vi "Robot Global Data.vi"() -> ()   [LabVIEW 2011]
doc: "This global VI can contain as many global variables as you need. Place a control on the panel, give it a good name. To read or write to it from a VI, drag the icon to the diagram of that VI. You can also drag from the project. Click on the node to change which global you access. You shouldn't have multiple locations writing to a global or it will cause a race-condition."
uses:
  <vilib>/Rock Robotics/WPI/Camera/WPI_CameraImageSize.ctl
panel:
  out "AUTO ON":bool
  out "is in auto":bool
  out "Target Locked":bool
  in  "Xerror":dbl=0.1
  in  "AUTO ON int":u8
  in  "teleop on":u8
  in  "Selected Distance":dbl
  in  "Distance":dbl
  in  "Elevator Button Prev":u8
  in  "Elevator Toggle":u8
  in  "LED toggle rate (ms)":u32=20
  in  "image size":T1=enum."320x240"
  in  "Enable Vision":bool
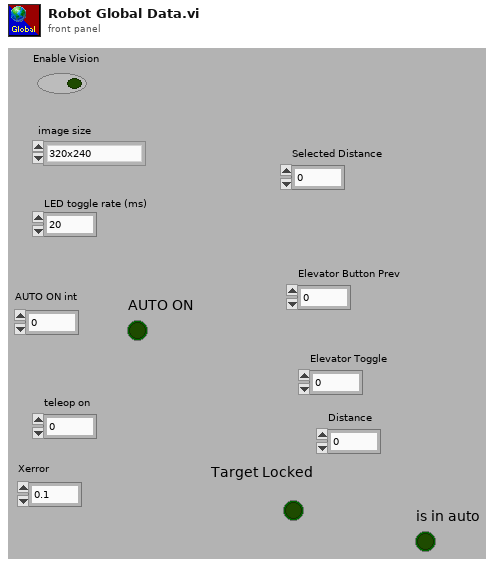
[diagram p1: front panel]
types:
  T1 = typedef "WPI_CameraImageSize.ctl" = enum16{"640x480", "320x240", "160x120"}
diagram:
